vi "nanocal -- nuclear schottky goodness V5.vi"(5 "action":T1=enum."onlygrads", 6 "parameters IN":map{T2, dbl}(c390), 7 "weighting strategy":T3, 8 "dz/dω IN (V)":cdb[](array[numeric])=[1.7183506006211996e-05+0.0i, 1.7124360968751133e-05+0.0i, 1.7049104347380084e-05+0.0i, 1.700437896335042e-05+0.0i, 1.6984579723285106e-05+0.0i, 1.702277369054923e-05+0.0i, 1.713094025845651e-05+0.0i, 1.734249707866828e-05+0.0i, 1.768320429215342e-05+0.0i, 1.8195281152538477e-05+0.0i, 1.8917228661806973e-05+0.0i, 1.9897834564883332e-05+0.0i, 2.154104046962704e-05+0.0i, 2.3247799321765792e-05+0.0i, 2.5364678450551808e-05+0.0i, 2.8645788781885885e-05+0.0i, 3.204749554800641e-05+0.0i, 3.783559691555022e-05+0.0i, 4.245015867332296e-05+0.0i, 4.909131821431355e-05+0.0i, 5.511821898441184e-05+0.0i, 6.178843506022867e-05+0.0i, 7.1079604965352e-05+0.0i, 7.922304381453334e-05+0.0i, 8.814778883893872e-05+0.0i, 9.806709148886077e-05+0.0i, 0.00011119043245647465+0.0i, 0.00012253184919712196+0.0i, 0.00013777724317049346+0.0i, 0.0001508081004573332+0.0i, 0.00016547294918783876+0.0i, 0.00018003847596605868+0.0i, 0.00019518361086534857+0.0i, 0.00021134179818259658+0.0i, 0.0002372041782935464+0.0i, 0.00025518143132024254+0.0i, 0.0002835129702467886+0.0i, 0.0003060118087631287+0.0i, 0.00032860772064336976+0.0i, 0.0003492674091322389+0.0i, 0.00037498324855458583+0.0i, 0.00040021078021115026+0.0i, 0.00041969942568205823+0.0i, 0.00044367338947118773+0.0i, 0.0004634793607238068+0.0i, 0.00047921028781215815+0.0i, 0.0004880906353641744+0.0i, 0.0004932212623741357+0.0i, 0.000491476456593048+0.0i, 0.000480893803992059+0.0i, 0.0004535995818650303+0.0i, 0.000417087772881063+0.0i, 0.0003564148692854789+0.0i, 0.0003049201646356487+0.0i, 0.00021260191240459413+0.0i, 0.00011714858948470126+0.0i, 1.675457544365132e-05+0.0i, -6.8674075405897e-05+0.0i, -0.000156473047607305+0.0i, -0.00026709373934749337+0.0i, -0.0003544271565676041+0.0i, -0.00047937600197311275+0.0i, -0.0006086290582260493+0.0i, -0.0007031877411848573+0.0i, -0.0007564526901441745+0.0i, -0.000802489180995596+0.0i, -0.0008414596018105983+0.0i, -0.0008809346482248761+0.0i, -0.0009073902840241921+0.0i, -0.0009264953054508651+0.0i, -0.0009405659412141811+0.0i, -0.000951649722530156+0.0i, -0.0009557485581057351+0.0i, -0.0009558464741053665+0.0i, -0.0009509110176922098+0.0i, -0.0009411315169847015+0.0i, -0.0009303400913929496+0.0i, -0.0009171113529290538+0.0i, -0.0009022111527275027+0.0i, -0.0008813746494947608+0.0i, -0.0008581837971946129+0.0i, -0.0008372063466683705+0.0i, -0.0008165626610594428+0.0i, -0.0007901155435838691+0.0i, -0.0007682834352800848+0.0i, -0.000746231015527196+0.0i, -0.0007238798463130141+0.0i, -0.0007015567569177018+0.0i, -0.000679301954671598+0.0i, -0.0006572001413831251+0.0i, -0.000629855254567978+0.0i, -0.0006083942229188815+0.0i, -0.0005768631156754208+0.0i, -0.0005562177438951648+0.0i, -0.0005359092039599222+0.0i, -0.0005145186443378148+0.0i, -0.0004951602053444319+0.0i, -0.00047624970229075174+0.0i, -0.0004577401041527736+0.0i, -0.00043519037796120065+0.0i], 9 "Voltage IN (V)":cdb[](array[numeric])=[1.7183506006211996e-05+0.0i, 1.7124360968751133e-05+0.0i, 1.7049104347380084e-05+0.0i, 1.700437896335042e-05+0.0i, 1.6984579723285106e-05+0.0i, 1.702277369054923e-05+0.0i, 1.713094025845651e-05+0.0i, 1.734249707866828e-05+0.0i, 1.768320429215342e-05+0.0i, 1.8195281152538477e-05+0.0i, 1.8917228661806973e-05+0.0i, 1.9897834564883332e-05+0.0i, 2.154104046962704e-05+0.0i, 2.3247799321765792e-05+0.0i, 2.5364678450551808e-05+0.0i, 2.8645788781885885e-05+0.0i, 3.204749554800641e-05+0.0i, 3.783559691555022e-05+0.0i, 4.245015867332296e-05+0.0i, 4.909131821431355e-05+0.0i, 5.511821898441184e-05+0.0i, 6.178843506022867e-05+0.0i, 7.1079604965352e-05+0.0i, 7.922304381453334e-05+0.0i, 8.814778883893872e-05+0.0i, 9.806709148886077e-05+0.0i, 0.00011119043245647465+0.0i, 0.00012253184919712196+0.0i, 0.00013777724317049346+0.0i, 0.0001508081004573332+0.0i, 0.00016547294918783876+0.0i, 0.00018003847596605868+0.0i, 0.00019518361086534857+0.0i, 0.00021134179818259658+0.0i, 0.0002372041782935464+0.0i, 0.00025518143132024254+0.0i, 0.0002835129702467886+0.0i, 0.0003060118087631287+0.0i, 0.00032860772064336976+0.0i, 0.0003492674091322389+0.0i, 0.00037498324855458583+0.0i, 0.00040021078021115026+0.0i, 0.00041969942568205823+0.0i, 0.00044367338947118773+0.0i, 0.0004634793607238068+0.0i, 0.00047921028781215815+0.0i, 0.0004880906353641744+0.0i, 0.0004932212623741357+0.0i, 0.000491476456593048+0.0i, 0.000480893803992059+0.0i, 0.0004535995818650303+0.0i, 0.000417087772881063+0.0i, 0.0003564148692854789+0.0i, 0.0003049201646356487+0.0i, 0.00021260191240459413+0.0i, 0.00011714858948470126+0.0i, 1.675457544365132e-05+0.0i, -6.8674075405897e-05+0.0i, -0.000156473047607305+0.0i, -0.00026709373934749337+0.0i, -0.0003544271565676041+0.0i, -0.00047937600197311275+0.0i, -0.0006086290582260493+0.0i, -0.0007031877411848573+0.0i, -0.0007564526901441745+0.0i, -0.000802489180995596+0.0i, -0.0008414596018105983+0.0i, -0.0008809346482248761+0.0i, -0.0009073902840241921+0.0i, -0.0009264953054508651+0.0i, -0.0009405659412141811+0.0i, -0.000951649722530156+0.0i, -0.0009557485581057351+0.0i, -0.0009558464741053665+0.0i, -0.0009509110176922098+0.0i, -0.0009411315169847015+0.0i, -0.0009303400913929496+0.0i, -0.0009171113529290538+0.0i, -0.0009022111527275027+0.0i, -0.0008813746494947608+0.0i, -0.0008581837971946129+0.0i, -0.0008372063466683705+0.0i, -0.0008165626610594428+0.0i, -0.0007901155435838691+0.0i, -0.0007682834352800848+0.0i, -0.000746231015527196+0.0i, -0.0007238798463130141+0.0i, -0.0007015567569177018+0.0i, -0.000679301954671598+0.0i, -0.0006572001413831251+0.0i, -0.000629855254567978+0.0i, -0.0006083942229188815+0.0i, -0.0005768631156754208+0.0i, -0.0005562177438951648+0.0i, -0.0005359092039599222+0.0i, -0.0005145186443378148+0.0i, -0.0004951602053444319+0.0i, -0.00047624970229075174+0.0i, -0.0004577401041527736+0.0i, -0.00043519037796120065+0.0i], 10 "ω (rad/sec)":dbl[](array[numeric])=[32012.991918577427, 32390.261658505893, 32466.39798177853, 32499.14340521798, 32517.39286113775, 32529.046092051318, 32537.14525712326, 32543.111142615544, 32547.696343954158, 32551.33675949651, 32554.302325209504, 32556.769142360055, 32558.856995237307, 32560.650202739795, 32562.209843476354, 32563.58125099723, 32564.7987833122, 32565.88895894197, 32566.872575330308, 32567.766175404246, 32568.583086316496, 32569.334166794306, 32570.02835688638, 32570.673085530187, 32571.274580490695, 32571.838104118455, 32572.36813539066, 32572.868514009202, 32573.342552524307, 32573.793126289274, 32574.222746575288, 32574.633618125405, 32575.027687968828, 32575.40668442971, 32575.772149741057, 32576.12546690325, 32576.467883345118, 32576.800529469096, 32577.124435064776, 32577.440543590797, 32577.749724325146, 32578.052781957467, 32578.35046682089, 32578.643482565894, 32578.932492128843, 32579.218126471686, 32579.500987779396, 32579.781656707495, 32580.06069600583, 32580.338656060805, 32580.616078519142, 32580.89350097748, 32581.171461032456, 32581.45050033079, 32581.73116925889, 32582.0140305666, 32582.29966469628, 32582.58867447239, 32582.88169000423, 32583.179375080817, 32583.48243271314, 32583.791613234323, 32584.10772197351, 32584.43162756919, 32584.764273480003, 32585.106690135035, 32585.460007297228, 32585.825472395412, 32586.204468856296, 32586.59853891288, 32587.009410462997, 32587.439030535847, 32587.889604513977, 32588.363642815923, 32588.86402143446, 32589.39405291983, 32589.957576334426, 32590.559071508098, 32591.203800151903, 32591.897990030815, 32592.64907072179, 32593.46598163404, 32594.359581707977, 32595.343197883154, 32596.433373726086, 32597.650906041054, 32599.022313348767, 32600.58195429849, 32602.375161800977, 32604.46301467823, 32606.929831615616, 32609.895397541775, 32613.535812870963, 32618.12101442274, 32624.086899701866, 32632.186064986967, 32643.839295900536, 32662.088751820305, 32694.834175046595, 32770.97049853239]) -> (0 "R norm":dbl=-1.0, 1 "G":dbl=-1.0, 2 "R(ω) out":cdb[](array[numeric])=[1.7183506006211996e-05+0.0i, 1.7124360968751133e-05+0.0i, 1.7049104347380084e-05+0.0i, 1.700437896335042e-05+0.0i, 1.6984579723285106e-05+0.0i, 1.702277369054923e-05+0.0i, 1.713094025845651e-05+0.0i, 1.734249707866828e-05+0.0i, 1.768320429215342e-05+0.0i, 1.8195281152538477e-05+0.0i, 1.8917228661806973e-05+0.0i, 1.9897834564883332e-05+0.0i, 2.154104046962704e-05+0.0i, 2.3247799321765792e-05+0.0i, 2.5364678450551808e-05+0.0i, 2.8645788781885885e-05+0.0i, 3.204749554800641e-05+0.0i, 3.783559691555022e-05+0.0i, 4.245015867332296e-05+0.0i, 4.909131821431355e-05+0.0i, 5.511821898441184e-05+0.0i, 6.178843506022867e-05+0.0i, 7.1079604965352e-05+0.0i, 7.922304381453334e-05+0.0i, 8.814778883893872e-05+0.0i, 9.806709148886077e-05+0.0i, 0.00011119043245647465+0.0i, 0.00012253184919712196+0.0i, 0.00013777724317049346+0.0i, 0.0001508081004573332+0.0i, 0.00016547294918783876+0.0i, 0.00018003847596605868+0.0i, 0.00019518361086534857+0.0i, 0.00021134179818259658+0.0i, 0.0002372041782935464+0.0i, 0.00025518143132024254+0.0i, 0.0002835129702467886+0.0i, 0.0003060118087631287+0.0i, 0.00032860772064336976+0.0i, 0.0003492674091322389+0.0i, 0.00037498324855458583+0.0i, 0.00040021078021115026+0.0i, 0.00041969942568205823+0.0i, 0.00044367338947118773+0.0i, 0.0004634793607238068+0.0i, 0.00047921028781215815+0.0i, 0.0004880906353641744+0.0i, 0.0004932212623741357+0.0i, 0.000491476456593048+0.0i, 0.000480893803992059+0.0i, 0.0004535995818650303+0.0i, 0.000417087772881063+0.0i, 0.0003564148692854789+0.0i, 0.0003049201646356487+0.0i, 0.00021260191240459413+0.0i, 0.00011714858948470126+0.0i, 1.675457544365132e-05+0.0i, -6.8674075405897e-05+0.0i, -0.000156473047607305+0.0i, -0.00026709373934749337+0.0i, -0.0003544271565676041+0.0i, -0.00047937600197311275+0.0i, -0.0006086290582260493+0.0i, -0.0007031877411848573+0.0i, -0.0007564526901441745+0.0i, -0.000802489180995596+0.0i, -0.0008414596018105983+0.0i, -0.0008809346482248761+0.0i, -0.0009073902840241921+0.0i, -0.0009264953054508651+0.0i, -0.0009405659412141811+0.0i, -0.000951649722530156+0.0i, -0.0009557485581057351+0.0i, -0.0009558464741053665+0.0i, -0.0009509110176922098+0.0i, -0.0009411315169847015+0.0i, -0.0009303400913929496+0.0i, -0.0009171113529290538+0.0i, -0.0009022111527275027+0.0i, -0.0008813746494947608+0.0i, -0.0008581837971946129+0.0i, -0.0008372063466683705+0.0i, -0.0008165626610594428+0.0i, -0.0007901155435838691+0.0i, -0.0007682834352800848+0.0i, -0.000746231015527196+0.0i, -0.0007238798463130141+0.0i, -0.0007015567569177018+0.0i, -0.000679301954671598+0.0i, -0.0006572001413831251+0.0i, -0.000629855254567978+0.0i, -0.0006083942229188815+0.0i, -0.0005768631156754208+0.0i, -0.0005562177438951648+0.0i, -0.0005359092039599222+0.0i, -0.0005145186443378148+0.0i, -0.0004951602053444319+0.0i, -0.00047624970229075174+0.0i, -0.0004577401041527736+0.0i, -0.00043519037796120065+0.0i], 3 "dG / d log α   OUT":map{T2, dbl}(c390))   [LabVIEW 2020]
uses:
  nanocal-goodness-weighting-strategy.ctl
  3-lorentzian-parameters.ctl
  3-lorentzian-heat-response action.ctl
  <vilib>/Utility/miscctls.llb/LVMapReplaceAction.ctl
  <vilib>/Analysis/_algsub.llb/Matrix Norm Type.ctl
  <vilib>/Analysis/baseanly.llb/Matrix Type of Inverse Matrix.ctl
  <vilib>/Analysis/baseanly.llb/Real A x B.vi
  <vilib>/Analysis/_algsub.llb/Real Matrix Norm.vi
  <vilib>/Analysis/Matrix/Numeric/Conversions/Array To Matrix - RA2.vi
  <vilib>/Analysis/baseanly.llb/Real Inverse Matrix.vi
  <vilib>/Analysis/Matrix/Numeric/Conversions/Array To Matrix - RA.vi
  <vilib>/Analysis/Matrix/Numeric/Conversions/Matrix To Array - RM.vi
  <vilib>/Analysis/Matrix/NI_Matrix.lvlib
  <vilib>/Analysis/NI_AALBase.lvlib
  <vilib>/Analysis/NI_AALPro.lvlib
panel:
  out "Real 2D Array":dbl[][](array[numeric])
  out "Array":dbl[][](array[numeric])
  out "d2G / d log α d log  β  matrix OUT":dbl[](array[numeric])
  out "d2G / d log α d log  β  map  OUT":map{i32[], dbl}(c390)
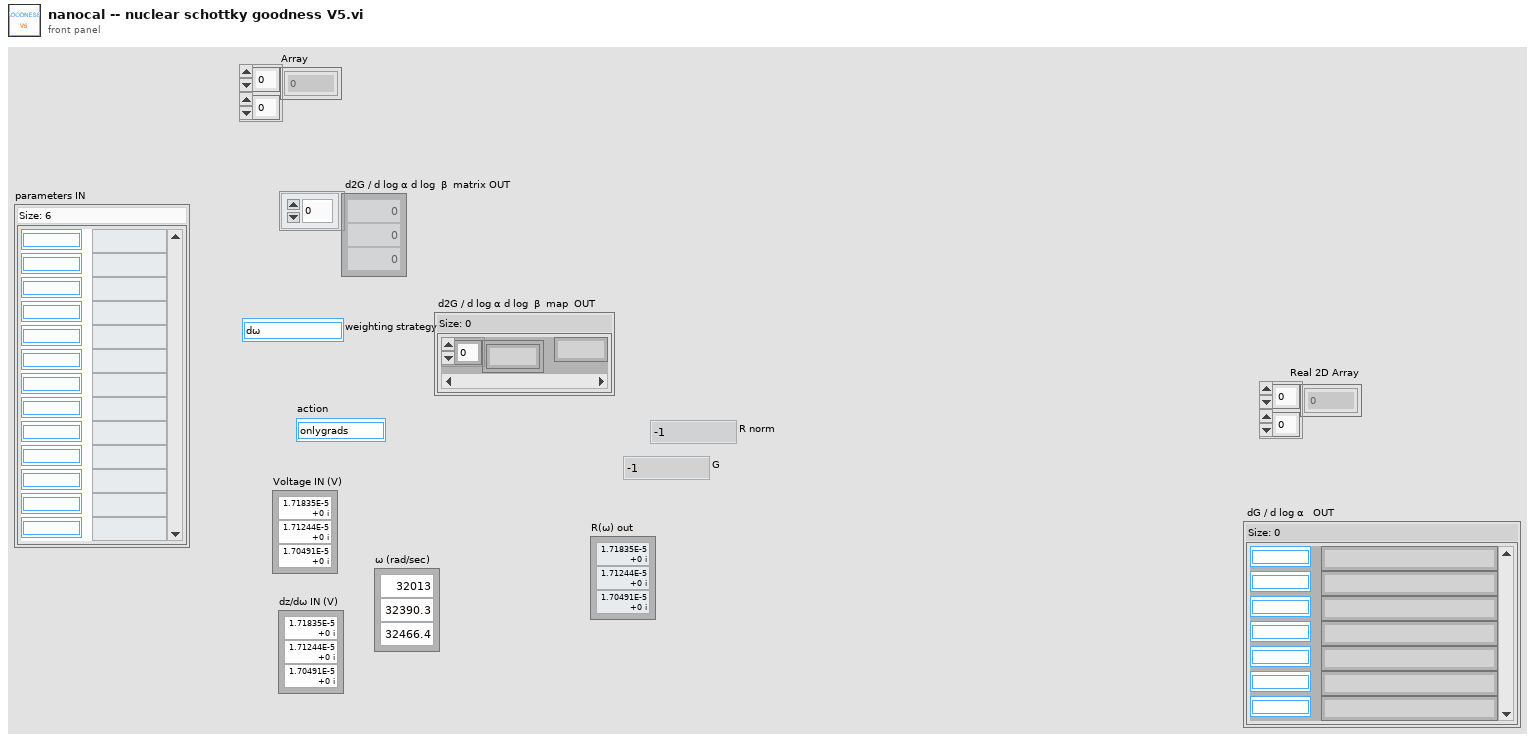
[diagram p1: front panel]
types:
  T1 = typedef "3-lorentzian-heat-response action.ctl" = enum16{"calc R", "create string", "calc m1m2m3", "dζ", "dT1", "dτS", "dτN", "dτC", "d-all", "dκ0", "T(K)", "m1", "m2", "m3", "parse string", "θ (deg)", "B (T)", "onlygrads", "newton", "create emty string"}
  T2 = typedef "3-lorentzian-parameters.ctl" = enum16{"ζ", "τ1", "τS", "τN", "τC", "κ0", "m1", "m2", "m3", "T (K)", "B (T)", "θ (deg)", "side (S|R)", "change (B|T)"}
  T3 = typedef "nanocal-goodness-weighting-strategy.ctl" = enum16{"dω", "dω √(|dz/dω|)", "dω |dz/dω|", "phase", "andreas", "sum"}
  T4 = typedef "LVMapReplaceAction.ctl" = enum32{"Modify Entry only if found", "Add or Modify Entry", "Delete Entry"}
  T5 = typedef "NI_AALBase.lvlib/Matrix Type of Inverse Matrix.ctl" = enum32{"General", "Positive Definite", "Lower Triangular", "Upper Triangular"}
  T6 = typedef "NI_AALPro.lvlib/Matrix Norm Type.ctl" = i32
  T7 = typedef "NI_Matrix.lvlib/RealMatrix.ctl" = dbl[][]
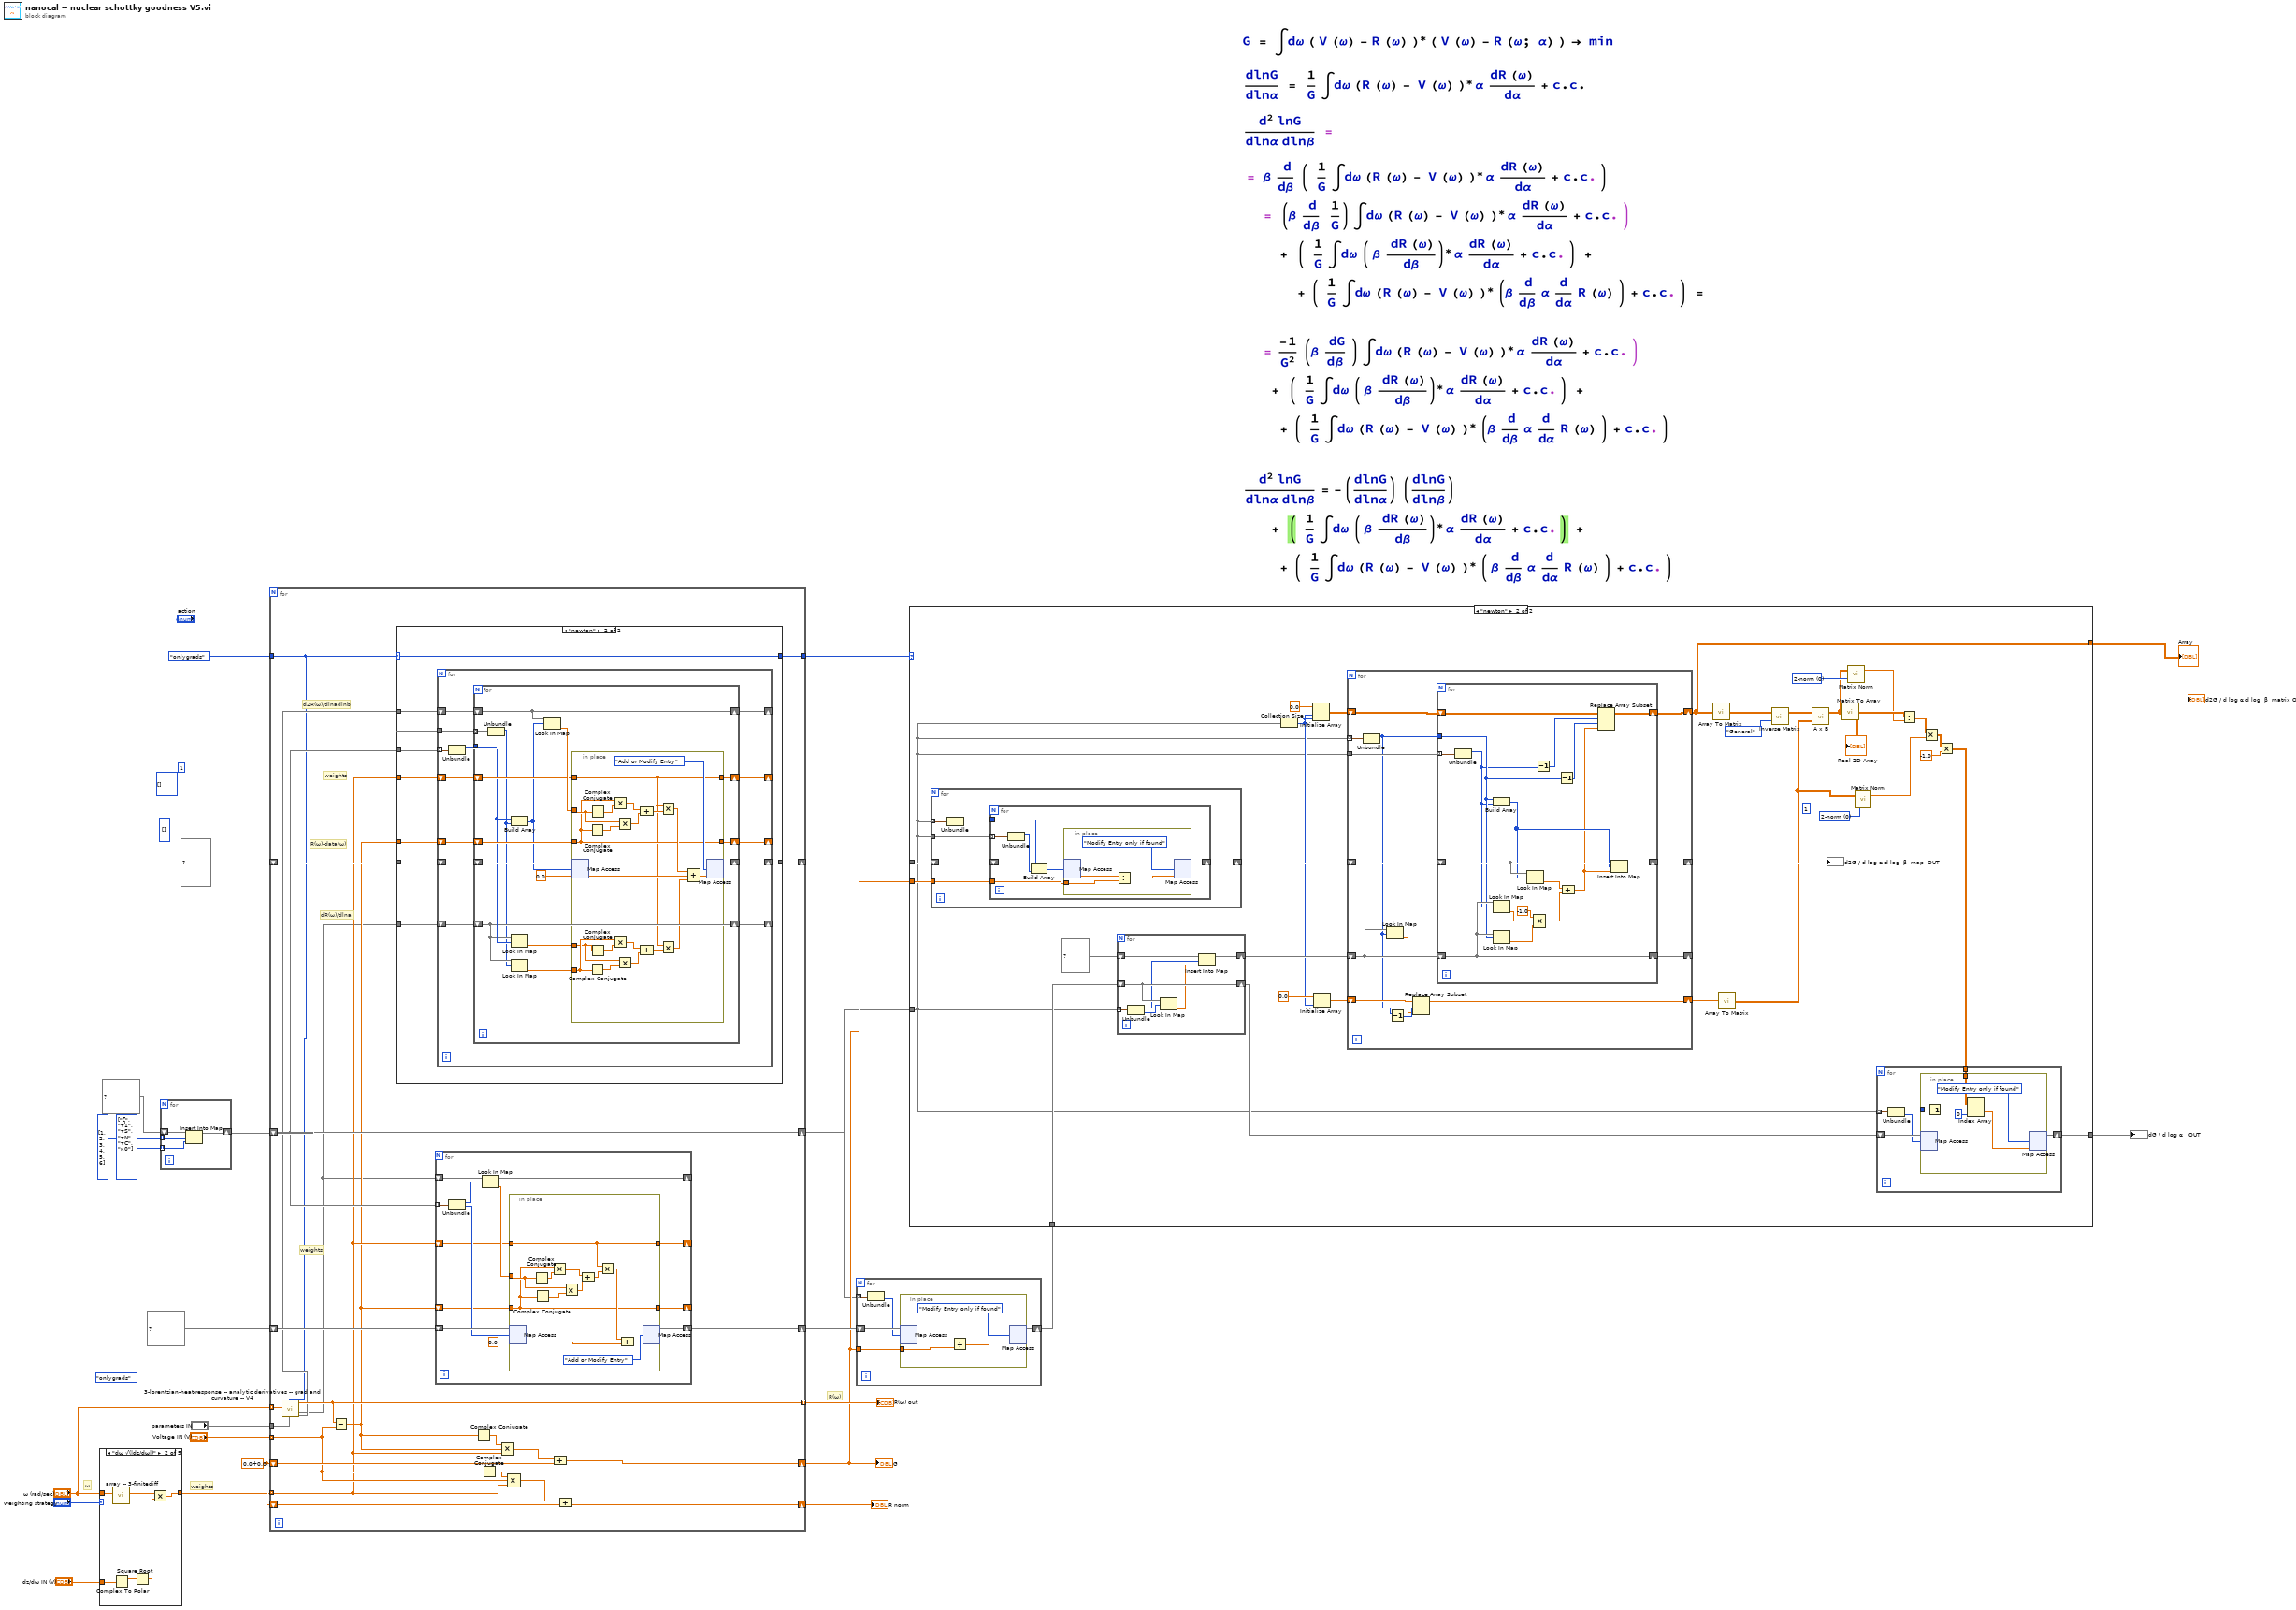
[diagram p0: block diagram]
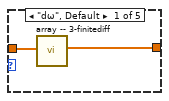
[diagram p3: hidden frame]
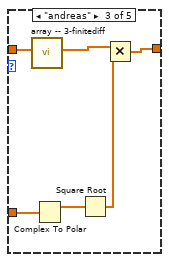
[diagram p4: hidden frame]
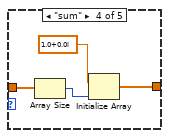
[diagram p5: hidden frame]
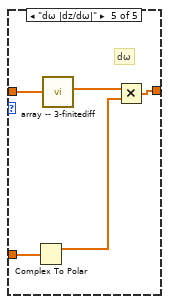
[diagram p6: hidden frame]
diagram:
  (unwired) 3-lorentzian-heat-response_action."onlygrads" ("action")
  (unwired) 1 ("index")
  (unwired) T2[] [] items=["ζ", "τ1", "τS", "τN", "τC", "κ0", "m1", "m2", "m3", "T (K)", "B (T)", "θ (deg)", "side (S|R)", "change (B|T)"]
  (unwired) i32[] []
  w14 = cdb 0.0+0.0i ("y")
  w19 = T2[] [enum."ζ", enum."τ1", enum."τS", enum."τN", enum."τC", enum."κ0"] items=["ζ", "τ1", "τS", "τN", "τC", "κ0", "m1", "m2", "m3", "T (K)", "B (T)", "θ (deg)", "side (S|R)", "change (B|T)"]
  # "weights"
  # "R(ω)"
  # "ω"
  n1 = case shown="\"dω √(|dz/dω|)\"" "weighting strategy" {
    tunnel: "dz/dω IN (V)" -> [_ w32 w38 _ w47]
    tunnel: "ω (rad/sec)" -> [w26 w28 w34 w42 w46]
    tunnel: [w25 w27 w33 w39 w43] -> w1
    frame "dω", Default {
      n2 = call "array -- 3-finitediff.vi"("ω (rad/sec)"=w26) -> ("dω (rad/sec)"=w25:cdb[])  [unwired: 10 in]
    }
    frame "dω √(|dz/dω|)" {
      n3 = call "array -- 3-finitediff.vi"("ω (rad/sec)"=w28) -> ("dω (rad/sec)"=w30:cdb[])  [unwired: 10 in]
      n4 = Complex To Polar(r * e^(i*theta)=w32) -> (r=w31:dbl[])  [unwired: 1 out]
      n5 = Square Root(x=w31) -> (sqrt(x)=w29:dbl[])
      n6 = Multiply(x=w30, y=w29) -> (x*y=w27:cdb[])
    }
    frame "andreas" {
      n7 = call "array -- 3-finitediff.vi"("ω (rad/sec)"=w34) -> ("dω (rad/sec)"=w36:cdb[])  [unwired: 10 in]
      n8 = Complex To Polar(r * e^(i*theta)=w38) -> (r=w37:dbl[])  [unwired: 1 out]
      n9 = Square Root(x=w37) -> (sqrt(x)=w35:dbl[])
      n10 = Multiply(x=w36, y=w35) -> (x*y=w33:cdb[])
    }
    frame "sum" {
      n11 = Array Size(array=w42) -> (size(s)=w41:i32)
      n12 = Initialize Array(cdb 1.0+0.0i ("y"), w41) -> (w39:cdb[])
    }
    frame "dω |dz/dω|" {
      # "dω"
      n13 = Complex To Polar(r * e^(i*theta)=w47) -> (r=w45:dbl[])  [unwired: 1 out]
      n14 = call "array -- 3-finitediff.vi"("ω (rad/sec)"=w46) -> ("dω (rad/sec)"=w44:cdb[])  [unwired: 10 in]
      n15 = Multiply(x=w44, y=w45) -> (x*y=w43:cdb[])
    }
  }
  n16 = for {
    tunnel: w19 -> [w48] mode=indexing
    shift-right: [w50] -> w12
    shift-left: map{i32, T2} {} ("parameters IN") -> [w51]
    tunnel: i32[] [1, 2, 3, 4, 5, 6] -> [w49] mode=indexing
    n17 = Insert Into Map(map in=w51, key=w49, value=w48) -> (map out=w50:map{i32, T2})  [unwired: 2 out]
  }
  n18 = for {
    tunnel: "ω (rad/sec)" -> [w73] mode=indexing
    tunnel: [w72] -> w21 mode=indexing
    tunnel: "parameters IN" -> [w74]
    tunnel: "Voltage IN (V)" -> [w61] mode=indexing
    tunnel: w1 -> [w56] mode=indexing
    shift-right: [w70] -> w15
    shift-left: map{T2, dbl} {} ("parameters IN") -> [w71]
    shift-right: [w60] -> w6
    shift-left: w12 -> [w60]
    shift-right: [w66] -> w8
    shift-left: w14 -> [w67]
    shift-right: [w62] -> w13
    shift-left: w14 -> [w63]
    shift-right: [w57] -> w9
    shift-left: map{i32[], dbl} {} ("parameters IN") -> [w58]
    tunnel: 3-lorentzian-heat-response_action."onlygrads" ("action") -> [w53]
    tunnel: [w52] -> w3
    # "R(ω)-data(ω)"
    # "weights"
    # "dR(ω)/dlna"
    # "d2R(ω)/dlnadlnb"
    # "weights"
    n19 = call "3-lorentzian-heat-response -- analytic derivatives -- grad and curvature -- V4.vi"("parameters map  IN"=w74, "action"=w53, "ω (rad/sec)"=w73) -> ("second derivatives map out"=w59:map{i32[], cdb}, "grad map  out"=w54:map{i32, cdb}, "R(ω)"=w72:cdb)  [unwired: 5 in, 1 out]
    n20 = Subtract(x=w72, y=w61) -> (x-y=w55:cdb)
    n21 = case shown="\"newton\"" w53 {
      selector: w53 -> [w75 w77]
      tunnel: w60 -> [_ w84]
      tunnel: w59 -> [_ w83]
      tunnel: w58 -> [w76 w82]
      tunnel: [w76 w81] -> w57
      tunnel: w56 -> [_ w80]
      tunnel: w55 -> [_ w79]
      tunnel: w54 -> [_ w78]
      tunnel: [w75 w77] -> w52
      frame "calc R", Default {
      }
      frame "newton" {
        n22 = for {
          shift-right: [w97] -> w81
          shift-left: w82 -> [w96]
          shift-right: [w95] -> _
          shift-left: w80 -> [w93]
          shift-right: [w94] -> _
          shift-left: w79 -> [w92]
          shift-right: [w91] -> _
          shift-left: w83 -> [w90]
          tunnel: w84 -> [w89] mode=indexing
          tunnel: w84 -> [w88]
          shift-right: [w85] -> _
          shift-left: w78 -> [w86]
          n23 = Unbundle(w89) -> ("index"=w87:i32)  [unwired: 1 out]
          n24 = for {
            shift-right: [w113] -> w91
            shift-left: w90 -> [w113]
            shift-right: [w110] -> w94
            shift-left: w92 -> [w109]
            shift-right: [w107] -> w97
            shift-left: w96 -> [w112]
            tunnel: w88 -> [w104] mode=indexing
            shift-right: [w105] -> w95
            shift-left: w93 -> [w106]
            tunnel: w87 -> [w102]
            shift-right: [w101] -> w85
            shift-left: w86 -> [w101]
            n25 = Unbundle(w104) -> ("index"=w100:i32)  [unwired: 1 out]
            n26 = Look In Map(map=w101, key=w100) -> (value=w98:cdb)  [unwired: 1 in, 1 out]
            n27 = Build Array(w102, w100) -> (w103:i32[])
            n28 = Look In Map(map=w101, key=w102) -> (value=w99:cdb)  [unwired: 1 in, 1 out]
            n29 = Look In Map(map=w113, key=w103) -> (value=w108:cdb)  [unwired: 1 in, 1 out]
            n30 = in-place {
              in-place-border: [w123] -> w110
              in-place-border: w109 -> [w123]
              in-place-border: w108 -> [w130]
              in-place-border: w106 -> [w115]
              in-place-border: [w115] -> w105
              in-place-border: w99 -> [w116]
              in-place-border: w98 -> [w117]
              n31 = in-place-map #1(w112, w103, 0.0 ("number")) -> (w129:dbl)  [unwired: 1 out]
              n32 = Complex Conjugate(1:w123) -> (0:w131:cdb)
              n33 = Complex Conjugate(1:w117) -> (0:w121:cdb)
              n34 = Complex Conjugate(1:w130) -> (0:w132:cdb)
              n35 = Complex Conjugate(1:w116) -> (0:w122:cdb)
              n36 = Multiply(x=w123, y=w132) -> (x*y=w127:cdb)
              n37 = Multiply(x=w117, y=w122) -> (x*y=w120:cdb)
              n38 = Multiply(x=w130, y=w131) -> (x*y=w126:cdb)
              n39 = Multiply(x=w116, y=w121) -> (x*y=w119:cdb)
              n40 = Compound Arithmetic op=ADD(w127, w126) -> (w125:cdb)
              n41 = Compound Arithmetic op=ADD(w120, w119) -> (w118:cdb)
              n42 = Multiply(x=w115, y=w125) -> (x*y=w124:cdb)
              n43 = Multiply(x=w115, y=w118) -> (x*y=w114:cdb)
              n44 = Compound Arithmetic op=ADD(w124, w129, w114) -> (w128:cdb)
              n45 = in-place-map #1(w128, LVMapReplaceAction."Add or Modify Entry" ("action")) -> (w107:map{i32[], dbl})  [unwired: 2 out]
            }
          }
        }
      }
    }
    n46 = for {
      shift-right: [w145] -> _
      shift-left: w54 -> [w145]
      shift-right: [w139] -> _
      shift-left: w55 -> [w138]
      shift-right: [w136] -> w70
      shift-left: w71 -> [w142]
      tunnel: w60 -> [w144] mode=indexing
      shift-right: [w134] -> _
      shift-left: w56 -> [w135]
      n47 = Unbundle(w144) -> ("index"=w143:i32, "X selector"=w141:T2)
      n48 = Look In Map(map=w145, key=w143) -> (value=w137:cdb)  [unwired: 1 in, 1 out]
      n49 = in-place {
        in-place-border: [w147] -> w139
        in-place-border: w138 -> [w147]
        in-place-border: w137 -> [w154]
        in-place-border: w135 -> [w146]
        in-place-border: [w146] -> w134
        n50 = in-place-map #2(w142, w141, 0.0 ("number")) -> (w153:dbl)  [unwired: 1 out]
        n51 = Complex Conjugate(1:w154) -> (0:w156:cdb)
        n52 = Complex Conjugate(1:w147) -> (0:w155:cdb)
        n53 = Multiply(x=w147, y=w156) -> (x*y=w151:cdb)
        n54 = Multiply(x=w154, y=w155) -> (x*y=w150:cdb)
        n55 = Compound Arithmetic op=ADD(w151, w150) -> (w149:cdb)
        n56 = Multiply(x=w146, y=w149) -> (x*y=w148:cdb)
        n57 = Compound Arithmetic op=ADD(w148, w153) -> (w152:cdb)
        n58 = in-place-map #2(w152, LVMapReplaceAction."Add or Modify Entry" ("action")) -> (w136:map{T2, dbl})  [unwired: 2 out]
      }
    }
    n59 = Complex Conjugate(1:w55) -> (0:w69:cdb)
    n60 = Complex Conjugate(1:w61) -> (0:w65:cdb)
    n61 = Compound Arithmetic op=MULTIPLY(w69, w55, w56) -> (w68:cdb)
    n62 = Compound Arithmetic op=MULTIPLY(w65, w61, w56) -> (w64:cdb)
    n63 = Compound Arithmetic op=ADD(w68, w67) -> (w66:cdb)
    n64 = Compound Arithmetic op=ADD(w64, w63) -> (w62:cdb)
  }
  "G" <- w8
  "R norm" <- w13
  "R(ω) out" <- w21
  n65 = for {
    tunnel: w6 -> [w159] mode=indexing
    shift-right: [w161] -> w10
    shift-left: w15 -> [w162]
    tunnel: w8 -> [w160]
    n66 = Unbundle(w159) -> ("X selector"=w158:T2)  [unwired: 1 out]
    n67 = in-place {
      in-place-border: w160 -> [w165]
      n68 = in-place-map #3(w162, w158) -> (w166:dbl)  [unwired: 1 in, 1 out]
      n69 = Divide(x=w166, y=w165) -> (x/y=w164:cdb)
      n70 = in-place-map #3(w164, LVMapReplaceAction."Modify Entry only if found" ("action")) -> (w161:map{T2, dbl})  [unwired: 2 out]
    }
  }
  n71 = case shown="\"newton\"" w3 {
    tunnel: w10 -> [w167 w197]
    tunnel: w9 -> [_ w196]
    tunnel: w8 -> [_ w194]
    tunnel: [_ w187] -> w7
    tunnel: w6 -> [_ w176]
    tunnel: [w167 w175] -> w5
    frame "calc R", Default {
    }
    frame "newton" {
      w182 = T6 0 items=["2-norm", "1-norm", "F-norm", "Inf-norm"] ("norm type")
      w183 = T6 0 items=["2-norm", "1-norm", "F-norm", "Inf-norm"] ("norm type")
      (unwired) 1 ("number of columns")
      n72 = for {
        tunnel: w176 -> [w215] mode=indexing
        tunnel: w176 -> [w216]
        shift-right: [w212] -> w195
        shift-left: w196 -> [w213]
        tunnel: w194 -> [w211]
        n73 = Unbundle(w215) -> ("index"=w214:i32)  [unwired: 1 out]
        n74 = for {
          tunnel: w216 -> [w223] mode=indexing
          tunnel: w214 -> [w222]
          shift-right: [w219] -> w212
          shift-left: w213 -> [w220]
          tunnel: w211 -> [w217]
          n75 = Unbundle(w223) -> ("index"=w221:i32)  [unwired: 1 out]
          n76 = Build Array(w222, w221) -> (w218:i32[])
          n77 = in-place {
            in-place-border: w217 -> [w226]
            n78 = in-place-map #4(w220, w218) -> (w227:dbl)  [unwired: 1 in, 1 out]
            n79 = Divide(x=w227, y=w226) -> (x/y=w225:cdb)
            n80 = in-place-map #4(w225, LVMapReplaceAction."Modify Entry only if found" ("action")) -> (w219:map{i32[], dbl})  [unwired: 2 out]
          }
        }
      }
      n81 = for {
        shift-right: [w263] -> w193
        shift-left: map{i32, dbl} {} ("parameters IN") -> [w264]
        tunnel: w176 -> [w262] mode=indexing
        shift-right: [w261] -> w177
        shift-left: w197 -> [w261]
        n82 = Unbundle(w262) -> ("index"=w259:i32, "X selector"=w260:T2)
        n83 = Look In Map(map=w261, key=w260) -> (value=w258:dbl)  [unwired: 1 in, 1 out]
        n84 = Insert Into Map(map in=w264, key=w259, value=w258) -> (map out=w263:map{i32, dbl})  [unwired: 2 out]
      }
      n85 = Collection Size(1:w176) -> (0:w184:i32)
      n86 = Initialize Array(0.0 ("number"), w184, w184) -> (w188:dbl[][])
      n87 = Initialize Array(0.0 ("number"), w184) -> (w191:dbl[])
      n88 = for {
        tunnel: w176 -> [w239] mode=indexing
        tunnel: w176 -> [w240]
        shift-right: [w237] -> w185
        shift-left: w195 -> [w238]
        shift-right: [w236] -> _
        shift-left: w193 -> [w234]
        shift-right: [w230] -> w189
        shift-left: w191 -> [w235]
        shift-right: [w229] -> w187
        shift-left: w188 -> [w228]
        n89 = Unbundle(w239) -> ("index"=w233:i32)  [unwired: 1 out]
        n90 = Look In Map(map=w234, key=w233) -> (value=w231:dbl)  [unwired: 1 in, 1 out]
        n91 = Decrement(x=w233) -> (x-1=w232:i32)
        n92 = Replace Array Subset(array=w235, new element=w231, index=w232) -> (w230:dbl[])
        n93 = for {
          tunnel: w240 -> [w257] mode=indexing
          tunnel: w233 -> [w245]
          shift-right: [w249] -> w237
          shift-left: w238 -> [w250]
          shift-right: [w256] -> w236
          shift-left: w234 -> [w256]
          shift-right: [w246] -> w229
          shift-left: w228 -> [w247]
          n94 = Unbundle(w257) -> ("index"=w244:i32)  [unwired: 1 out]
          n95 = Build Array(w245, w244) -> (w248:i32[])
          n96 = Look In Map(map=w256, key=w244) -> (value=w254:dbl)  [unwired: 1 in, 1 out]
          n97 = Look In Map(map=w256, key=w245) -> (value=w255:dbl)  [unwired: 1 in, 1 out]
          n98 = Look In Map(map=w250, key=w248) -> (value=w252:dbl)  [unwired: 1 in, 1 out]
          n99 = Compound Arithmetic op=MULTIPLY(-1.0 ("value"), w254, w255) -> (w251:dbl)
          n100 = Decrement(x=w244) -> (x-1=w243:i32)
          n101 = Decrement(x=w245) -> (x-1=w242:i32)
          n102 = Compound Arithmetic op=ADD(w252, w251) -> (w241:dbl)
          n103 = Replace Array Subset(array=w247, new element=w241, index (row)=w243, index (col)=w242) -> (w246:dbl[][])
          n104 = Insert Into Map(map in=w250, key=w248, value=w241) -> (map out=w249:map{i32[], dbl})  [unwired: 2 out]
        }
      }
      "d2G / d log α d log  β  map  OUT" <- w185
      n105 = call-poly <vilib>:"Array To Matrix.vi"("Real 2D Array"=w187) -> ("Real Matrix"=w171:T7)
      n106 = call-poly <vilib>:"Array To Matrix.vi"("Real 1D Array"=w189) -> ("Real Matrix (Column Vector)"=w168:T7)
      n107 = call-poly <vilib>:"Inverse Matrix.vi"("matrix type"=Matrix_Type_of_Inverse_Matrix."General", "Input Matrix"=w171) -> ("Inverse Matrix"=w170:T7)  [unwired: 1 out]
      n108 = call-poly <vilib>:"A x B.vi"("B"=w168, "A"=w170) -> ("A x B"=w169:T7)  [unwired: 1 out]
      n109 = call-poly <vilib>:"Matrix To Array.vi"("Real Matrix"=w169) -> ("Real 2D Array"=w181:dbl[][])
      "Real 2D Array" <- w181
      n110 = call-poly <vilib>:"Matrix Norm.vi"("norm type"=w183, "Input Matrix"=w169) -> ("norm"=w180:dbl)  [unwired: 1 out]
      n111 = call-poly <vilib>:"Matrix Norm.vi"("norm type"=w182, "Input Matrix"=w168) -> ("norm"=w178:dbl)  [unwired: 1 out]
      n112 = Divide(x=w181, y=w180) -> (x/y=w179:dbl[][])
      n113 = Multiply(x=w179, y=w178) -> (x*y=w174:dbl[][])
      n114 = Multiply(x=w174, y=-1.0) -> (x*y=w172:dbl[][])
      n115 = for {
        tunnel: w176 -> [w202] mode=indexing
        shift-right: [w203] -> w175
        shift-left: w177 -> [w204]
        tunnel: w172 -> [w200]
        n116 = Unbundle(w202) -> ("index"=w199:i32, "X selector"=w201:T2)
        n117 = in-place {
          in-place-border: w200 -> [w209]
          in-place-border: w199 -> [w208]
          n118 = in-place-map #5(w204, w201) -> ()  [unwired: 1 in, 2 out]
          n119 = Decrement(x=w208) -> (x-1=w207:i32)
          n120 = Index Array(array=w209, index (row)=w207, index (col)=0 ("disabled index (col)")) -> (element=w206:dbl)
          n121 = in-place-map #5(w206, LVMapReplaceAction."Modify Entry only if found" ("action")) -> (w203:map{T2, dbl})  [unwired: 2 out]
        }
      }
    }
  }
  "dG / d log α   OUT" <- w5
  "Array" <- w7
